vi "Save File Load Dialog Data.vi"(8 "error in (no error)":errorcluster, 10 "FileDialog":T2={"File"=path "", "Group"="", "Channel"="", "DataPlugin"="", "MissingTeeth"=0.0, "ErrState"="", "File Selected"=FALSE, "Data Selection Method"=enum."Manual", "Offset"=0, "Length"=0, "DataPlugins Info"=[], "Controls"=[], "File Ref"=refnum, "Groups"=[], "Channels"=[], "Groups Refs"=[], "Channel Refs"=[], "Cancelled"=FALSE, "CycleAngle?"=FALSE, "FPGA memory size"=enum."32,768", "DAC Bits"=1, "GroupRef"=refnum, "ChanRef"=refnum, "Data"=[], "ReverseData"=FALSE} {"DAC Bits" min=1 max=16}, 11 "Node Ptr":T1 format="%.0x") -> (0 "error out":errorcluster)   [LabVIEW 2011, in "Engine Sim System Explorer.lvlib"]
uses:
  Engine Sim System Explorer.lvlib
  TypeDefs/File Load Dialog.ctl
  TypeDefs/Data Replay Data Selection Method.ctl
  <vilib>/Platform/storage/utility/usiPluginInformation.ctl
  TypeDefs/AngleReference.ctl
  TypeDefs/FPGA Mem Size.ctl
  <vilib>/NI Veristand/Custom Device API/Custom Device Item Ref.ctl
  Shared/Engine Simulation Global.vi
  <vilib>/NI Veristand/Custom Device API/Set Item Property (Boolean).vi
  <vilib>/NI Veristand/Custom Device API/Set Item Property (Dependent File).vi
  <vilib>/NI Veristand/Custom Device API/Set Item Property (String).vi
  <vilib>/NI Veristand/Custom Device API/Set Item Property (Double).vi
  <vilib>/NI Veristand/Custom Device API/Set Item Property (I32).vi
  Engine Simulation Shared.lvlib
  <vilib>/NI Veristand/Custom Device API/Custom Device API.lvlib
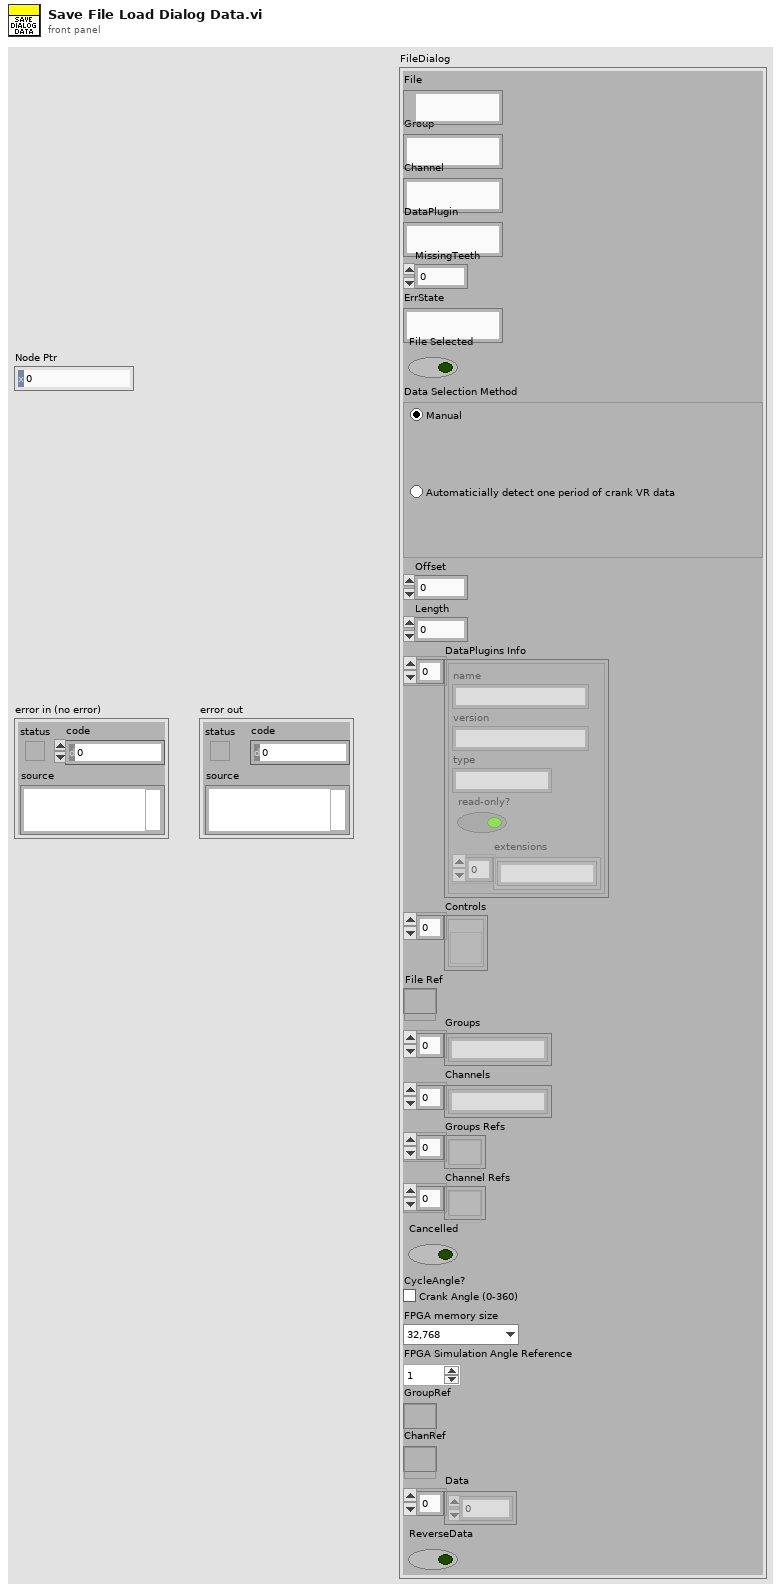
[diagram p1: front panel]
types:
  T1 = typedef "Custom Device API.lvlib/Custom Device Item Ref.ctl" = u64
  T2 = typedef "Engine Sim System Explorer.lvlib/File Load Dialog.ctl" = cluster{"File":path, "Group":string, "Channel":string, "DataPlugin":string, "MissingTeeth":dbl, "ErrState":string, "File Selected":bool, "Data Selection Method":T3, "Offset":i32, "Length":i32, "DataPlugins Info":T4[], "Controls":refnum<vi>[], "File Ref":refnum<k20>, "Groups":string[], "Channels":string[], "Groups Refs":refnum<k20>[], "Channel Refs":refnum<k20>[], "Cancelled":bool, "CycleAngle?":T5, "FPGA memory size":T6, "DAC Bits":u16, "GroupRef":refnum<k20>, "ChanRef":refnum<k20>, "Data":dbl[], "ReverseData":bool}
  T3 = typedef "Engine Sim System Explorer.lvlib/Data Replay Data Selection Method.ctl" = enum32{"Manual", "AutoVRCrank"}
  T4 = typedef "usiPluginInformation.ctl" = cluster{"name":string, "version":string, "type":string, "read-only?":bool, "extensions":string[]}
  T5 = typedef "Engine Sim System Explorer.lvlib/AngleReference.ctl" = bool
  T6 = typedef "Engine Sim System Explorer.lvlib/FPGA Mem Size.ctl" = enum16{"32,768", "16,384", "8,192", "4,096", "2,048", "1024", "512", "256", "128"}
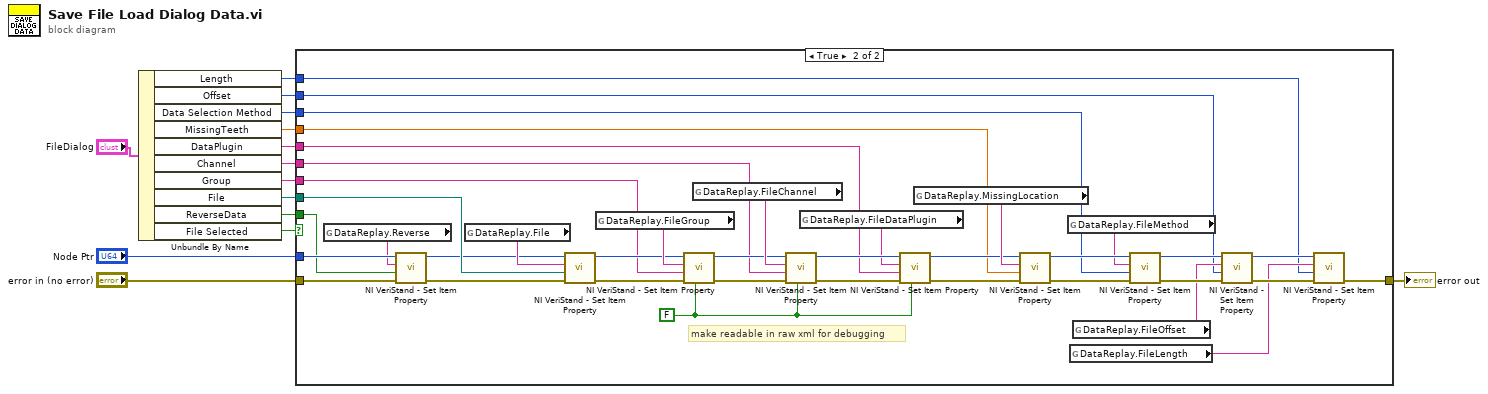
[diagram p0: block diagram]
diagram:
  n1 = Unbundle By Name("FileDialog") -> ("Length"=w2:i32, "Offset"=w3:i32, "Data Selection Method"=w4:T3, "MissingTeeth"=w5:dbl, "DataPlugin"=w6:string, "Channel"=w7:string, "Group"=w8:string, "File"=w9:path, "ReverseData"=w1:bool, "File Selected"=w10:bool)
  n2 = case shown="True" w10 {
    tunnel: "Node Ptr" -> [_ w19]
    tunnel: "error in (no error)" -> [w15 w31]
    tunnel: [w15 w36] -> w14
    tunnel: w9 -> [_ w29]
    tunnel: w8 -> [_ w28]
    tunnel: w7 -> [_ w27]
    tunnel: w6 -> [_ w26]
    tunnel: w5 -> [_ w25]
    tunnel: w4 -> [_ w24]
    tunnel: w3 -> [_ w23]
    tunnel: w2 -> [_ w22]
    tunnel: w1 -> [_ w16]
    frame False {
    }
    frame True {
      w21 = FALSE ("Binary String (T)")
      # "make readable in raw xml for debugging"
      n3 = global read "Engine Simulation Global.vi" "DataReplay.Reverse"() -> (w17:string)
      n4 = call-poly <vilib>:"NI VeriStand - Set Item Property.vi"("error in (no error)"=w31, "Value"=w16, "Property Name"=w17, "Item Ref in"=w19) -> ("error out"=w20:errorcluster, "Item Ref out"=w18:T1)  [unwired: 5 in, 1 out]
      n5 = global read "Engine Simulation Global.vi" "DataReplay.File"() -> (w30:string)
      n6 = call-poly <vilib>:"NI VeriStand - Set Item Property.vi"("error in (no error)"=w20, "Path"=w29, "Property Name"=w30, "Item Ref in"=w18) -> ("error out"=w32:errorcluster, "Item Ref out"=w33:T1)  [unwired: 5 in, 1 out]
      n7 = global read "Engine Simulation Global.vi" "DataReplay.FileGroup"() -> (w53:string)
      n8 = call-poly <vilib>:"NI VeriStand - Set Item Property.vi"("Binary String (T)"=w21, "error in (no error)"=w32, "Value"=w28, "Property Name"=w53, "Item Ref in"=w33) -> ("error out"=w50:errorcluster, "Item Ref out"=w51:T1)  [unwired: 4 in, 1 out]
      n9 = global read "Engine Simulation Global.vi" "DataReplay.FileChannel"() -> (w52:string)
      n10 = call-poly <vilib>:"NI VeriStand - Set Item Property.vi"("Binary String (T)"=w21, "error in (no error)"=w50, "Value"=w27, "Property Name"=w52, "Item Ref in"=w51) -> ("error out"=w48:errorcluster, "Item Ref out"=w49:T1)  [unwired: 4 in, 1 out]
      n11 = global read "Engine Simulation Global.vi" "DataReplay.FileDataPlugin"() -> (w47:string)
      n12 = call-poly <vilib>:"NI VeriStand - Set Item Property.vi"("Binary String (T)"=w21, "error in (no error)"=w48, "Value"=w26, "Property Name"=w47, "Item Ref in"=w49) -> ("error out"=w44:errorcluster, "Item Ref out"=w45:T1)  [unwired: 4 in, 1 out]
      n13 = global read "Engine Simulation Global.vi" "DataReplay.MissingLocation"() -> (w46:string)
      n14 = call-poly <vilib>:"NI VeriStand - Set Item Property.vi"("error in (no error)"=w44, "Value"=w25, "Property Name"=w46, "Item Ref in"=w45) -> ("error out"=w42:errorcluster, "Item Ref out"=w43:T1)  [unwired: 5 in, 1 out]
      n15 = global read "Engine Simulation Global.vi" "DataReplay.FileMethod"() -> (w41:string)
      n16 = global read "Engine Simulation Global.vi" "DataReplay.FileLength"() -> (w34:string)
      n17 = global read "Engine Simulation Global.vi" "DataReplay.FileOffset"() -> (w35:string)
      n18 = call-poly <vilib>:"NI VeriStand - Set Item Property.vi"("error in (no error)"=w42, "Value"=w24, "Property Name"=w41, "Item Ref in"=w43) -> ("error out"=w39:errorcluster, "Item Ref out"=w40:T1)  [unwired: 5 in, 1 out]
      n19 = call-poly <vilib>:"NI VeriStand - Set Item Property.vi"("error in (no error)"=w39, "Value"=w23, "Property Name"=w35, "Item Ref in"=w40) -> ("error out"=w37:errorcluster, "Item Ref out"=w38:T1)  [unwired: 5 in, 1 out]
      n20 = call-poly <vilib>:"NI VeriStand - Set Item Property.vi"("error in (no error)"=w37, "Value"=w22, "Property Name"=w34, "Item Ref in"=w38) -> ("error out"=w36:errorcluster)  [unwired: 5 in, 2 out]
    }
  }
  "error out" <- w14
